vi "SOUR_POW_CORR_COLL_FCH_STAT.vi"(0 "VISA IN":refnum<visa-resource-name>, 1 "Cal Frq. Checking ON/OFF":bool, 5 "error in":errorcluster, 7 "Channel":i32) -> (14 "VISA Out":refnum<visa-resource-name>, 19 "error out":errorcluster)   [LabVIEW 2018, in "PNA-X.lvlib"]
doc: "SOURce<cnum>:POWer:CORRection:COLLect:FCHeck[:STATe] <ON | OFF> \n(Read-Write) Enables and disables frequency checking of source power cal acquisition sweeps. \nONLY use when you have more than one power sensor. \nParameters \n<cnum> Any existing channel number. If unspecified, value is set to 1 \n<ON|OFF> ON (1) turns source power cal frequency checking ON. A requested \nacquisition will only succeed for those frequency points which fall within a \nfrequency range specified for the power sensor being used. An acquisition will \npause in mid-sweep if the frequency is about to exceed the maximum \nfrequency limit specified for that sensor. When the sweep is paused in this \nmanner, a sensor connected to the other channel input of the power meter can \nbe connected to the measurement port in place of the previous sensor, and used \nto complete the sweep. However, the maximum frequency specified for the \n1838\n\nsecond sensor would need to be sufficient for the sweep to complete. \nFrequency limits are specified using the SOUR:POW:CORR:COLL:SEN \ncommand. \nOFF (0) - turns source power cal frequency checking OFF. An acquisition will \nuse just one power sensor for the entire sweep, regardless of frequency. \nExamples SOUR:POW:CORR:COLL:FCH ON \nsource1:power2:correction:collect:fcheck:state off \nQuery Syntax SOURce:POWer:CORRection:COLLect:FCHeck[:STATe]? \nReturn Type Boolean (1 = ON, 0 = OFF) \nDefault OFF (0) \nSOURce:POWer:CORRection:COLLect:ITERation[:COUNt] <num> \n(Read-Write) This command, along with SOUR:POW:CORR:COLL:ITER:NTOL describes the \nnumber of ADUSTMENTS to make to the source power. \nSets the maximum number of readings to take at each data point for iterating the source power. Power \nREADINGS (performed by SOUR:POW:CORR:COLL:AVER:COUNT and \nSOUR:POW:CORR:COLL:AVER:NTOLerance) will continue to be made, and source power \nadjusted, until the measurement is within the iteration tolerance value or this max number of \nmeasurements has been met. The last value is the valid measurement for that data point. \nLearn more. \nParameters \n<num> Maximum number of readings. Choose any number between 1 and 100. \nExamples SOUR:POW:CORR:COLL:ITER 2 \nsource:power:correction:collect:iteration 3 \nQuery Syntax SOURce:POWer:CORRection:COLLect:ITERation[:COUNt]? \nReturn Type Numeric \nDefault 1 \nSOURce:POWer:CORRection:COLLect:ITERation:NTOLerance <num> \n1839\n\n(Read-Write) This command, along with SOUR:POW:CORR:COLL:ITER:COUNT describes the \nnumber of ADUSTMENTS to make to the source power. \nSets the maximum desired deviation from the sum of the test port power and the offset value. Power \nREADINGS (performed by SOUR:POW:CORR:COLL:AVER:COUNT and \nSOUR:POW:CORR:COLL:AVER:NTOLerance) will continue to be made, and source power \nadjusted, until a measurement is within this tolerance value or the max number of measurements has \nbeen met. The last value is the valid measurement for that data point. \nLearn more. \nParameters \n<cnum> Any existing channel number. If unspecified, value is set to 1 \n<port> Port number to correct for source power. If unspecified, value is set to 1. \n<num> Tolerance value in dBm. Choose any number between 0 and 5 \nExamples SOUR:POW:CORR:COLL:ITER:NTOL .005 \nsource:power:correction:collect:iteration:ntolerance .1 \nQuery Syntax SOURce:POWer:CORRection:COLLect:ITERation:NTOLerance? \nReturn Type Numeric \nDefault .05"
uses:
  PNA-X.lvlib
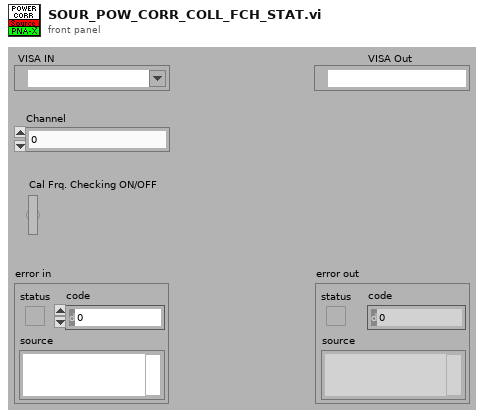
[diagram p1: front panel]
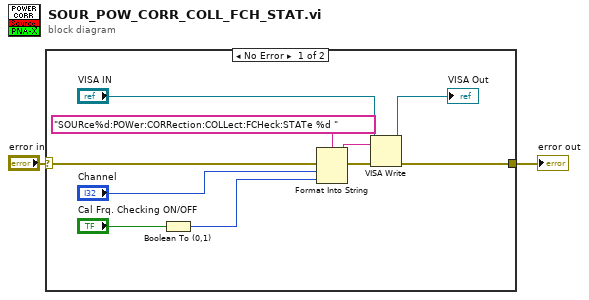
[diagram p0: block diagram]
diagram:
  n1 = case shown="No Error" "error in" {
    selector: "error in" -> [w12 w13]
    tunnel: [w7 w13] -> w1
    frame No Error {
      n2 = Boolean To (0,1)(Boolean="Cal Frq. Checking ON/OFF") -> (0, 1=w3:i16)
      n3 = Format Into String(format string="SOURce%d:POWer:CORRection:COLLect:FCHeck:STATe %d " ("Cmdline"), error in=w12, "Channel", w3) -> (resulting string=w10:string, error out=w11:errorcluster)  [unwired: 1 in]
      n4 = VISA Write(VISA resource name="VISA IN", write buffer=w10, error in (no error)=w11) -> (VISA resource name out=→"VISA Out":refnum<visa-resource-name>, error out=w7:errorcluster)  [unwired: 1 out]
    }
    frame Error {
    }
  }
  "error out" <- w1
